vi "simple caluclator.vi"() -> ()   [LabVIEW 2022 SP3]
panel:
  in  "stop":bool
  out "RESULT":dbl
  in  "DIV":bool
  in  "MUL":bool
  in  "Sub":bool
  in  "Add":bool
  in  "B":dbl
  in  "A":dbl
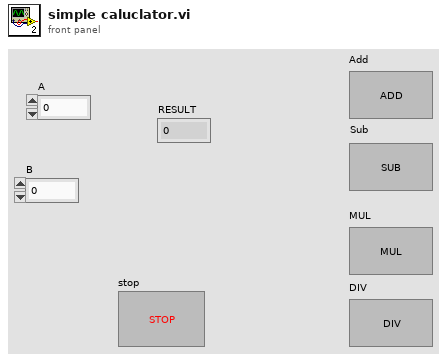
[diagram p1: front panel]
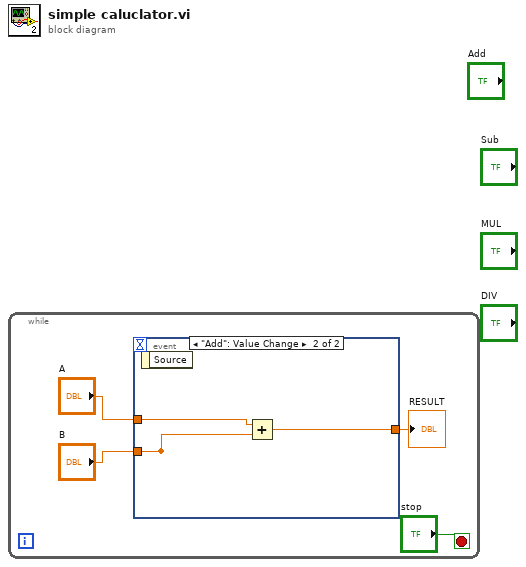
[diagram p0: block diagram]
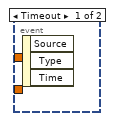
[diagram p2: hidden frame]
diagram:
  n1 = while {
    stop <- "stop" stop-if-true
    n2 = event shown="[1] \"Add\": Value Change" {
      selector: _ -> [_ _]
      dyn-events: _ -> [_ _]
      timeout: _ -> [_ _]
      tunnel: "A" -> [_ w7]
      tunnel: [_ w6] -> _
      tunnel: "B" -> [_ w6]
      tunnel: [_ w5] -> w2
      event Timeout {
        n3 = event-data() -> ()  [unwired: 1 in, 3 out]
      }
      event "Add": Value Change {
        n4 = event-data() -> ()  [unwired: 1 in, 1 out]
        n5 = Add(x=w7, y=w6) -> (x+y=w5:dbl)
      }
    }
    "RESULT" <- w2
  }
